vi "Tell Child.vi"(4 "Priority":bool, 6 "Alias":string, 7 "Actor in":refnum<class "Actor.lvclass">, 8 "Error in":errorcluster, 9 "Called From Msg Library":bool, 10 "Msg":refnum<class "Msg.lvclass">) -> (0 "Error out":errorcluster, 5 "Actor out":refnum<class "Actor.lvclass">)   [LabVIEW 2020, in "jettl.lvlib"]
uses:
  jettl.lvlib
  Msg/Msg.lvclass
  Actor/Actor.lvclass
  Relation.ctl
  Read Self Attributes/Read Self Attributes.lvlib
  Read Child Attributes/Read Child Attributes.lvlib
  Teller Elements.ctl
  Read Self Attributes/Alias.vi
  Read Child Attributes/Transport.vi
  Read Self Attributes/UID.vi
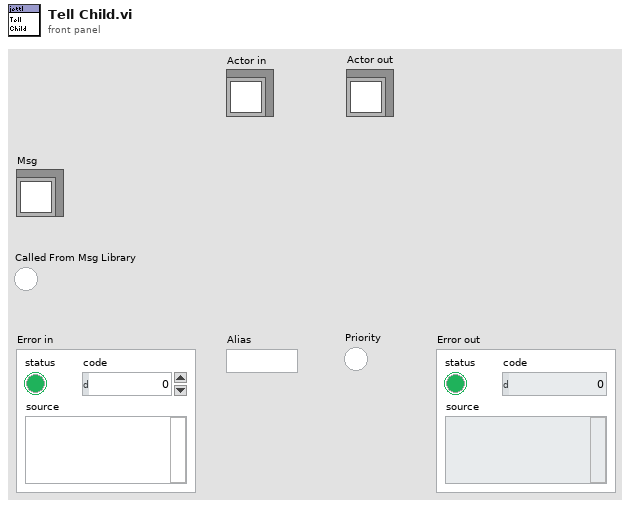
[diagram p1: front panel]
types:
  T1 = typedef "jettl.lvlib/Teller Elements.ctl" = cluster{"Priority":bool, "Relative Seconds":dbl, "UID":i32, "Alias":string, "Valid Relation":bool, "Relation":T2, "Called From Msg Library":bool}
  T2 = typedef "jettl.lvlib/Relation.ctl" = enum16{"Self", "Parent", "Child"}
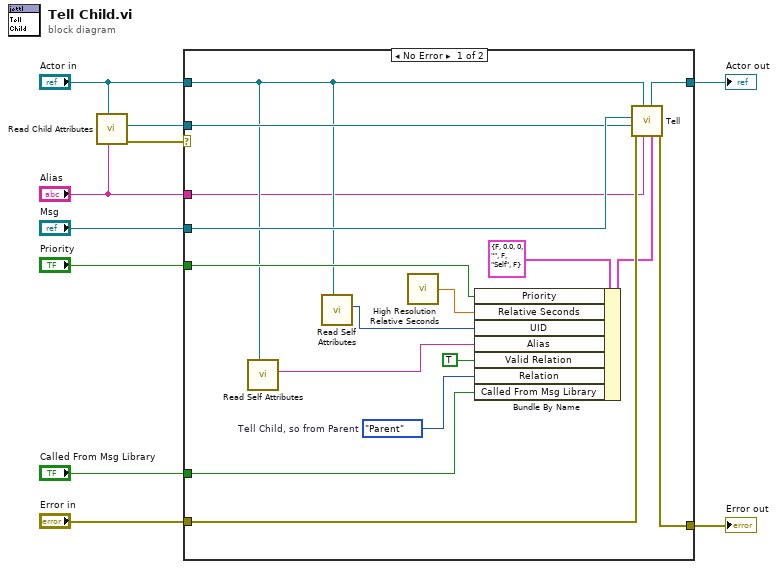
[diagram p0: block diagram]
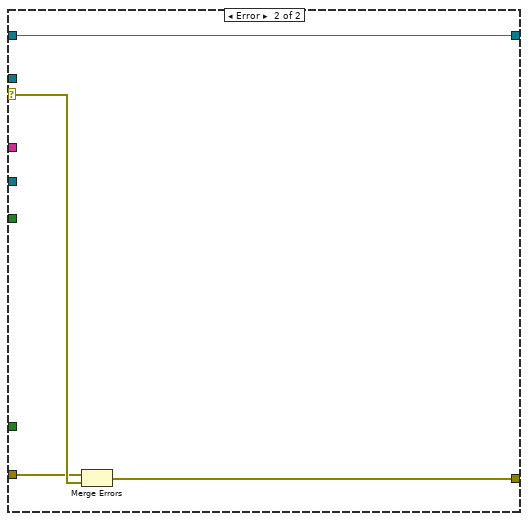
[diagram p2: hidden frame]
diagram:
  n1 = call-poly "Read Child Attributes.vi"("Alias"="Alias", "Actor in"="Actor in") -> ("Error out"=w4:errorcluster, "Transport"=w5:refnum<class "Transport.lvclass">)  [unwired: 8 in]
  n2 = case shown="No Error" w4 {
    selector: w4 -> [_ w29]
    tunnel: "Actor in" -> [w16 w27]
    tunnel: [w20 w27] -> w10
    tunnel: "Alias" -> [w11 _]
    tunnel: [w19 w30] -> w9
    tunnel: "Msg" -> [w22 _]
    tunnel: "Error in" -> [w26 w28]
    tunnel: w5 -> [w21 _]
    tunnel: "Priority" -> [w17 _]
    tunnel: "Called From Msg Library" -> [w23 _]
    frame No Error {
      w15 = Relation."Parent"  # Tell Child, so from Parent
      n3 = call-poly "Read Self Attributes.vi"("Actor in"=w16) -> ("Alias"=w14:string)  [unwired: 10 in]
      n4 = call-poly "Read Self Attributes.vi"("Actor in"=w16) -> ("UID"=w25:i32)  [unwired: 10 in]
      n5 = call <vilib>:"High Resolution Relative Seconds.vi"() -> ("relative seconds"=w18:dbl)
      n6 = Bundle By Name(cluster=T1 {"Priority"=FALSE, "Relative Seconds"=0.0, "UID"=0, "Alias"="", "Valid Relation"=FALSE, "Relation"=enum."Self", "Called From Msg Library"=FALSE} ("Teller Elements"), "Priority"=w17, "Relative Seconds"=w18, "UID"=w25, "Alias"=w14, "Valid Relation"=TRUE, "Relation"=w15, "Called From Msg Library"=w23) -> (w12:T1)
      n7 = call "Tell.vi"("Teller Elements"=w12, "Alias"=w11, "Actor in"=w16, "Error in"=w26, "Transport"=w21, "Msg"=w22) -> ("Error out"=w19:errorcluster, "Actor out"=w20:refnum<class "Actor.lvclass">)  [unwired: 4 in]
    }
    frame Error {
      n8 = Merge Errors(w28, w29) -> (w30:errorcluster)
    }
  }
  "Error out" <- w9
  "Actor out" <- w10
